vi "Load Image.vi"(8 "error in (no error)":errorcluster, 10 "Image Data":T1, 11 "Image File":path) -> (0 "error out":errorcluster, 3 "Image":refnum<k24>)   [LabVIEW 2013]
doc: "This VI will load an image file into a PictureBox .Net control. The file it will load is the one provided by <B>Image File</B>. It will then display the image using the setting found in <B>Size Mode (Zoom)</B>. Zoom will make the picture fit the control while keeping the aspect ratio, while Stretch will fill the control in all directions.\n\nIf a file is not provided by <B>Image File</B>, the data found in <B>Image Data</B> will be used instead to display the image into the PictureBox.\n\nNote that the image does not stay in the PictureBox after the VI has stopped executing.\n\n-----\nBrian Hoover (hooovahh)"
uses:
  <vilib>/picture/picture.llb/imagedata.ctl
  System.Drawing
  <vilib>/Utility/colorconv.llb/Color to RGB.vi
  <vilib>/wsapi/NI_WebServices.lvlib
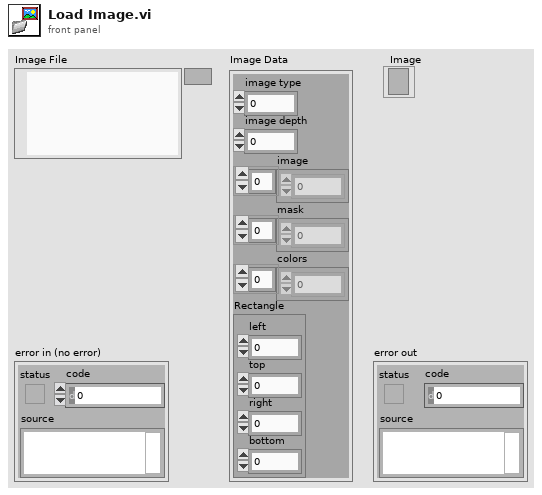
[diagram p1: front panel]
types:
  T1 = typedef "imagedata.ctl" = cluster{"image type":i32, "image depth":i32, "image":u8[], "mask":u8[], "colors":u32[], "Rectangle":cluster{"left":i16, "top":i16, "right":i16, "bottom":i16}}
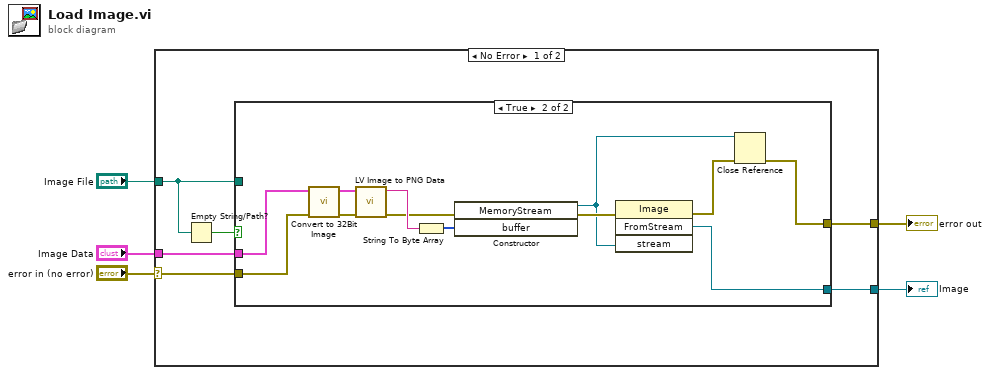
[diagram p0: block diagram]
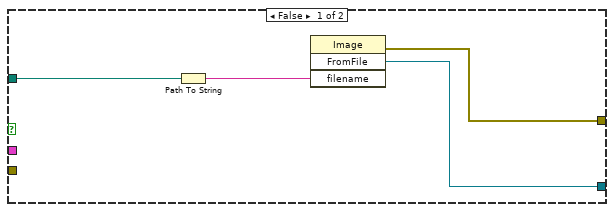
[diagram p2: hidden frame]
diagram:
  n1 = case shown="No Error" "error in (no error)" {
    selector: "error in (no error)" -> [w8 w28]
    tunnel: "Image Data" -> [w10 _]
    tunnel: "Image File" -> [w9 _]
    tunnel: [w7 _] -> w3
    tunnel: [w6 w28] -> w2
    frame No Error {
      n2 = Empty String/Path?(string/path=w9) -> (empty?=w11:bool)
      n3 = case shown="True" w11 {
        tunnel: w10 -> [_ w18]
        tunnel: w9 -> [w14 _]
        tunnel: w8 -> [_ w17]
        tunnel: [w15 w21] -> w7
        tunnel: [w12 w16] -> w6
        frame False {
          n4 = Path To String(path=w14) -> (string=w13:string)
          n5 = invoke class="Image" method="FromFile"("filename"=w13) -> (error out=w12:errorcluster, "FromFile"=w15:refnum<k24>)  [unwired: 3 in, 2 out]
        }
        frame True {
          n6 = call "Convert to 32Bit Image.vi"("error in (no error)"=w17, "Image Data"=w18) -> ("error out"=w26:errorcluster, "32Bit Image Data Out"=w27:T1)  [unwired: 8 in]
          n7 = call <vilib>:"LV Image to PNG Data.vi"("error in (no error)"=w26, "image data"=w27) -> ("error out"=w23:errorcluster, "png data"=w24:string)  [unwired: 8 in]
          n8 = String To Byte Array(string=w24) -> (unsigned byte array=w25:u8[])
          n9 = constructor class="MemoryStream"(error in=w23, "buffer"=w25) -> (reference out=w20:refnum<k24>, error out=w22:errorcluster)  [unwired: 2 in, 2 out]
          n10 = invoke class="Image" method="FromStream"(error in=w22, "stream"=w20) -> (error out=w19:errorcluster, "FromStream"=w21:refnum<k24>)  [unwired: 2 in, 2 out]
          n11 = Close Reference(reference=w20, error in (no error)=w19) -> (error out=w16:errorcluster)
        }
      }
    }
    frame Error {
    }
  }
  "error out" <- w2
  "Image" <- w3
